vi "daqio_Write_Waveform.vi"(6 "Waveform Info":string, 7 "daq.io Device Channel Key":string, 8 "error in (no error)":errorcluster, 10 "Waveform":waveform(dbl), 11 "daq.io type in":T1={"daq.io ref"=refnum, "daq.io API Base"="http://dashboard.daq.io/api/v1", "Device Key"="", "Account ID"="", "online"=TRUE, "SSL"=FALSE, "buffer"=TRUE}) -> (0 "error out":errorcluster, 3 "daq.io type out":T1={"daq.io ref"=refnum, "daq.io API Base"="http://dashboard.daq.io/api/v1", "Device Key"="", "Account ID"="", "online"=TRUE, "SSL"=FALSE, "buffer"=TRUE})   [LabVIEW 2013, in "daqio minimal.lvlib"]
doc: "This VI writes a waveform packet to a channel of a daq.io device. Wire a LabVIEW waveform type to this VI and it will be stored on daq.io. \n\nIf the daq.io Device Channel does not exist online, a new channel will be auto-created and data will be stored there. You have to provide a Channel Key where the value will be written to."
uses:
  daqio minimal.lvlib
  _typedefs/daqio-Type.ctl
  <vilib>/httpClient/ClientHandle.ctl
  _typedefs/daqio-WaveformEntry.ctl
  _typedefs/daqio-Buffer-Commands.ctl
  _typedefs/connection_FGV_commands.ctl
  <vilib>/Easy HTTP Client/Easy HTTP.lvlib
  <vilib>/httpClient/LabVIEWHTTPClient.lvlib
panel:
  out "JSON string":string
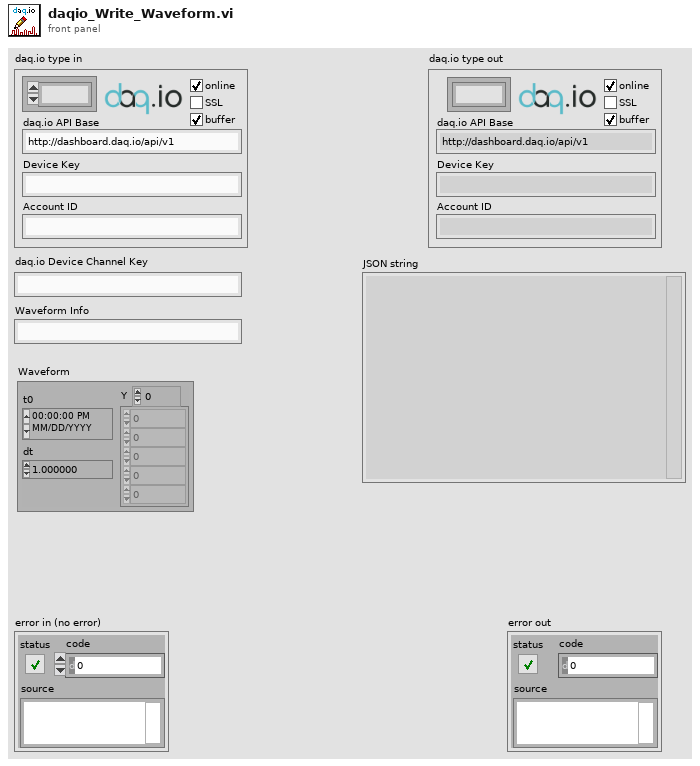
[diagram p1: front panel]
types:
  T1 = typedef "daqio minimal.lvlib/daqio-Type.ctl" = cluster{"daq.io ref":T2, "daq.io API Base":string, "Device Key":string, "Account ID":string, "online":bool, "SSL":bool, "buffer":bool}
  T2 = typedef "LabVIEWHTTPClient.lvlib/ClientHandle.ctl" = refnum<k1>
  T3 = typedef "daqio minimal.lvlib/daqio-WaveformEntry.ctl" = cluster{"device":string, "channel":string, "label":string, "start_time":string, "delta":dbl, "values":dbl[]}
  T4 = typedef "daqio minimal.lvlib/daqio-Buffer-Commands.ctl" = enum16{"Add to Buffer", "Post from Buffer", "Clear Buffer", "Init"}
  T5 = typedef "daqio minimal.lvlib/connection_FGV_commands.ctl" = enum16{"Set Conn Stat", "Save Key", "Get Key from File", "Set Type", "Set Buffer", "Get"}
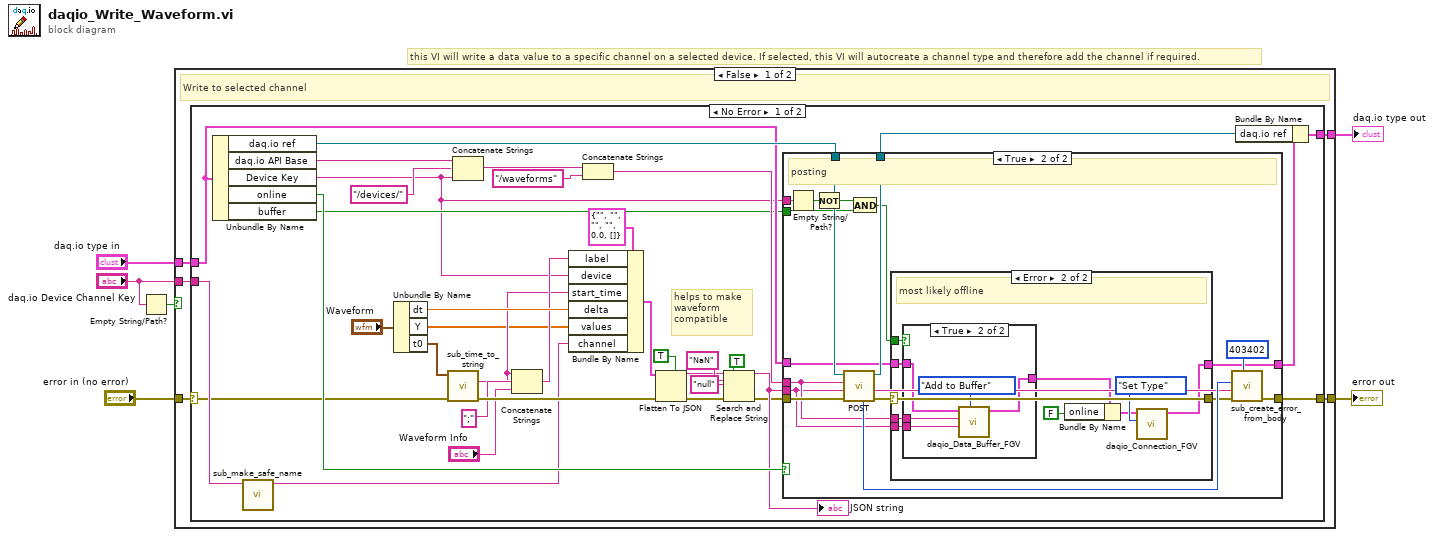
[diagram p0: block diagram]
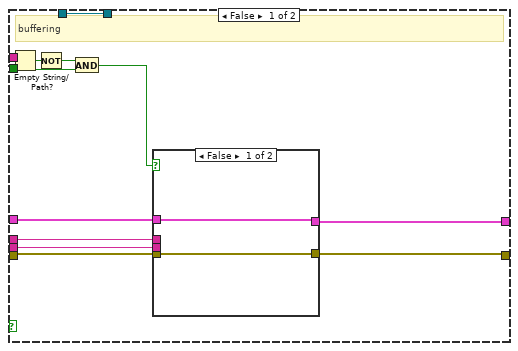
[diagram p2: hidden frame]
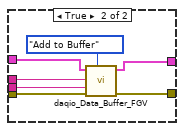
[diagram p3: hidden frame]
diagram:
  # "this VI will write a data value to a specific channel on a selected device. If selected, this VI will autocreate a channel type and therefore add the channel if required."
  n1 = Empty String/Path?(string/path="daq.io Device Channel Key") -> (empty?=w3:bool)
  n2 = case shown="False" w3 {
    tunnel: "daq.io type in" -> [w11 w108]
    tunnel: [w10 w108] -> w6
    tunnel: [w9 w107] -> w5
    tunnel: "error in (no error)" -> [w8 w107]
    tunnel: "daq.io Device Channel Key" -> [w7 _]
    frame False {
      # "Write to selected channel"
      n3 = case shown="No Error" w8 {
        selector: w8 -> [w24 w105]
        tunnel: w11 -> [w21 w106]
        tunnel: [w46 w106] -> w10
        tunnel: [w36 w105] -> w9
        tunnel: w7 -> [w38 _]
        frame No Error {
          # "helps to make \nwaveform\ncompatible"
          n4 = Unbundle By Name(w21) -> ("daq.io ref"=w40:T2, "daq.io API Base"=w45:string, "Device Key"=w19:string, "online"=w26:bool, "buffer"=w20:bool)
          n5 = call "sub_make_safe_name.vi"("Input String"=w38) -> ("Safe Output String"=w25:string)  [unwired: 10 in]
          n6 = Unbundle By Name("Waveform") -> ("dt"=w32:dbl, "Y"=w22:dbl[], "t0"=w23:timestamp)
          n7 = call "sub_time_to_string.vi"("error in (no error)"=w24, "timestamp"=w23) -> ("error out"=w37:errorcluster, "time"=w27:string)  [unwired: 8 in]
          n8 = Concatenate Strings(w45, "/devices/", w19) -> (w41:string)
          n9 = Concatenate Strings(w27, ";" ("string"), "Waveform Info") -> (w28:string)
          n10 = Bundle By Name(cluster=T3 {"device"="", "channel"="", "label"="", "start_time"="", "delta"=0.0, "values"=[]} ("Cluster"), "label"=w28, "device"=w19, "start_time"=w27, "delta"=w32, "values"=w22, "channel"=w25) -> (w47:T3)
          n11 = Concatenate Strings(w41, "/waveforms") -> (w42:string)
          n12 = Flatten To JSON(enable LabVIEW extensions? (T)=TRUE, anything=w47, error in (no error)=w37) -> (JSON string=w15:string, 11:w13:errorcluster)
          n13 = Search and Replace String(replace all?=TRUE ("replace all? (F)"), input string=w15, search string="NaN", replace string="null" ("replace string (\"\")"), error in=w13) -> (result string=w14:string, error out=w12:errorcluster)  [unwired: 3 in, 2 out]
          "JSON string" <- w14
          n14 = case shown="True" w26 {
            tunnel: w12 -> [w57 w86]
            tunnel: [w59 w85] -> w44
            tunnel: w42 -> [w54 w77]
            tunnel: w40 -> [w59 w84]
            tunnel: w14 -> [w56 w76]
            tunnel: [w58 w83] -> w36
            tunnel: [w55 w78] -> w35
            tunnel: w21 -> [w53 w74]
            tunnel: w20 -> [w49 w70]
            tunnel: w19 -> [w50 w71]
            frame False {
              # "buffering"
              n15 = Empty String/Path?(string/path=w50) -> (empty?=w51:bool)
              n16 = Not(x=w51) -> (.not. x?=w52:bool)
              n17 = And(x=w52, y=w49) -> (x .and. y?=w48:bool)
              n18 = case shown="False" w48 {
                tunnel: [w60 w68] -> w58
                tunnel: w57 -> [w60 w67]
                tunnel: w56 -> [_ w66]
                tunnel: [w61 w65] -> w55
                tunnel: w54 -> [_ w64]
                tunnel: w53 -> [w61 w62]
                frame False {
                }
                frame True {
                  n19 = call "daqio_Data_Buffer_FGV.vi"("Buffer Command"=daqio-Buffer-Commands."Add to Buffer", "error in (no error)"=w67, "JSON Data"=w66, "API route"=w64, "daq.io type in"=w62) -> ("error out"=w68:errorcluster, "daq.io type out"=w65:T1)  [unwired: 5 in]
                }
              }
            }
            frame True {
              # "posting"
              n20 = Empty String/Path?(string/path=w71) -> (empty?=w73:bool)
              n21 = Not(x=w73) -> (.not. x?=w72:bool)
              n22 = call <vilib>:"POST.vi"("error in (no error)"=w86, "data"=w76, "url"=w77, "client handle"=w84) -> ("error out"=w79:errorcluster, "body"=w80:string, "client handle out"=w85:T2, "HTTP Response Code"=w82:i32)  [unwired: 3 in, 1 out]
              n23 = And(x=w72, y=w70) -> (x .and. y?=w69:bool)
              n24 = case shown="Error" w79 {
                selector: w79 -> [w88 w98]
                tunnel: [w88 w98] -> w75
                tunnel: [w87 w93] -> w78
                tunnel: w77 -> [_ w92]
                tunnel: w76 -> [_ w91]
                tunnel: w74 -> [w87 w90]
                tunnel: w69 -> [_ w89]
                frame No Error {
                }
                frame Error {
                  # "most likely offline"
                  n25 = case shown="True" w89 {
                    tunnel: [w99 w103] -> w96
                    tunnel: w92 -> [_ w102]
                    tunnel: w91 -> [_ w101]
                    tunnel: w90 -> [w99 w100]
                    frame False {
                    }
                    frame True {
                      n26 = call "daqio_Data_Buffer_FGV.vi"("Buffer Command"=daqio-Buffer-Commands."Add to Buffer", "JSON Data"=w101, "API route"=w102, "daq.io type in"=w100) -> ("daq.io type out"=w103:T1)  [unwired: 6 in, 1 out]
                    }
                  }
                  n27 = Bundle By Name(cluster=w96, "online"=FALSE) -> (w94:T1)
                  n28 = call "daqio_Connection_FGV.vi"("Command"=connection_FGV_commands."Set Type" ("Enum"), "daq.io type in"=w94) -> ("daq.io type out"=w93:T1)  [unwired: 6 in, 3 out]
                }
              }
              n29 = call "sub_create_error_from_body.vi"("error code"=403402, "error in (no error)"=w75, "http code"=w82, "body"=w80) -> ("error out"=w83:errorcluster)  [unwired: 7 in]
            }
          }
          n30 = Bundle By Name(cluster=w35, "daq.io ref"=w44) -> (w46:T1)
        }
        frame Error {
        }
      }
    }
    frame True {
      # "no Channel Key: nothing to do"
    }
  }
  "error out" <- w5
  "daq.io type out" <- w6
